vi "S2C_IMAGE_Proc_Timed.vi"(8 "Error In":errorcluster, 10 "DisplayTime":dbl, 11 "ImagePath":path) -> (0 "Error Out":errorcluster)   [LabVIEW 2015]
panel:
  out "Image":picture
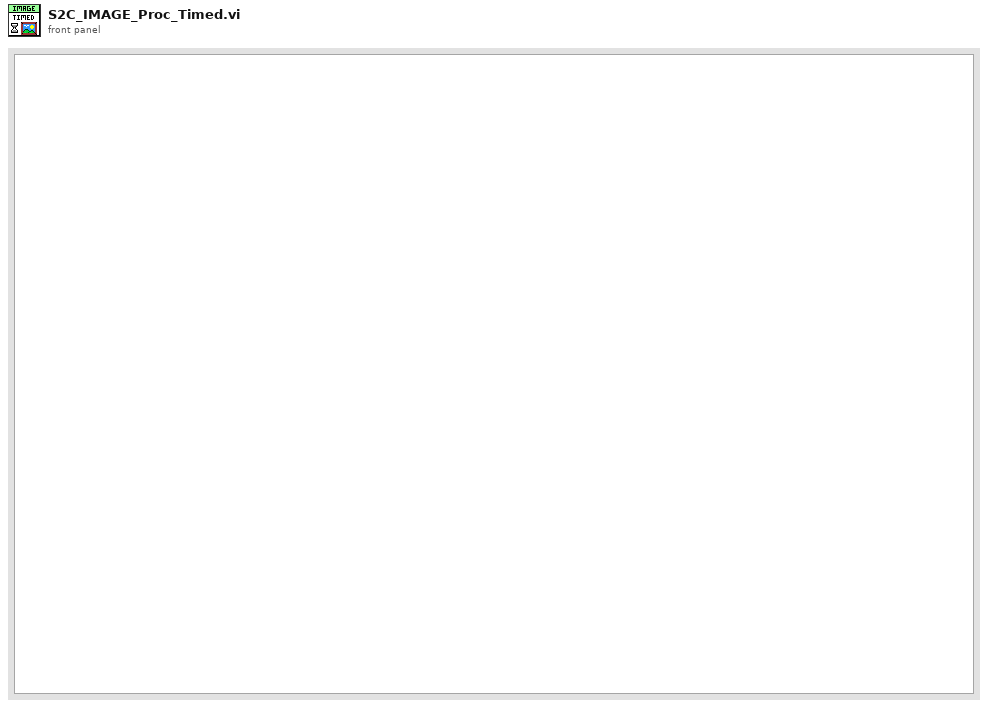
[diagram p1: front panel]
types:
  T1 = cluster{"Left":i16, "Top":i16, "Right":i16, "Bottom":i16}
  T2 = enum32{"Invalid", "Standard", "Closed", "Hidden", "Minimized", "Maximized"}
  T3 = typedef "imagedata.ctl" = cluster{"image type":i32, "image depth":i32, "image":u8[], "mask":u8[], "colors":u32[], "Rectangle":cluster{"left":i16, "top":i16, "right":i16, "bottom":i16}}
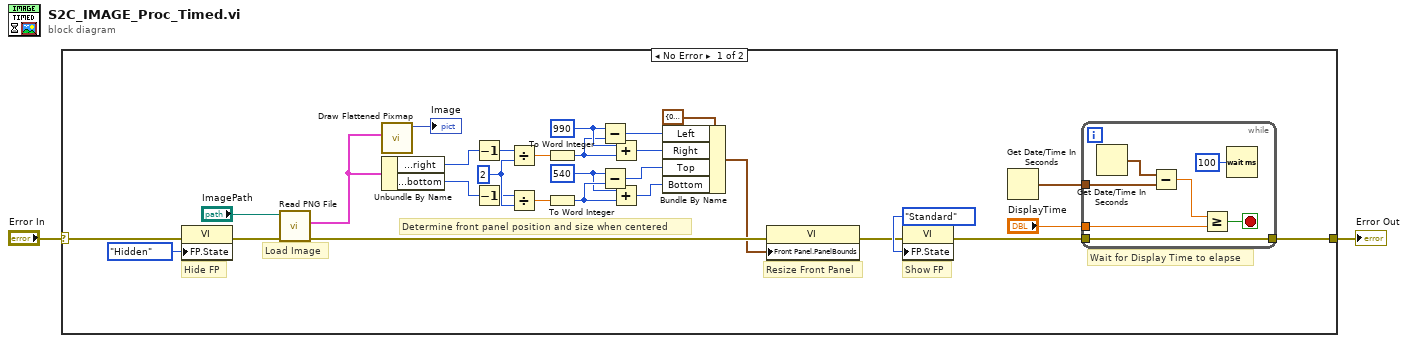
[diagram p0: block diagram]
diagram:
  n1 = case shown="No Error" "Error In" {
    selector: "Error In" -> [w26 w40]
    tunnel: [w30 w40] -> w1
    frame No Error {
      w13 = i16 540
      w16 = i16 990
      w20 = i16 2 ("y")
      # "Show FP"
      # "Resize Front Panel"
      # "Determine front panel position and size when centered"
      # "Hide FP"
      # "Wait for Display Time to elapse"
      # "Load Image"
      n2 = property class="VI"(error in=w26, "FP.State"=T2."Hidden" ("Front Panel Window:State")) -> (error out=w24:errorcluster)  [unwired: 1 in, 1 out]
      n3 = call <vilib>:"Read PNG File.vi"("error in (no error)"=w24, "path to PNG file"="ImagePath") -> ("error out"=w7:errorcluster, "image data"=w27:T3)  [unwired: 7 in, 1 out]
      n4 = call <vilib>:"Draw Flattened Pixmap.vi"("image data"=w27) -> ("new picture"=→"Image":picture)  [unwired: 8 in]
      n5 = Unbundle By Name(w27) -> ("Rectangle.right"=w17:i16, "Rectangle.bottom"=w19:i16)
      n6 = Decrement(x=w17) -> (x-1=w4:i16)
      n7 = Decrement(x=w19) -> (x-1=w3:i16)
      n8 = Divide(x=w4, y=w20) -> (x/y=w18:dbl)
      n9 = Divide(x=w3, y=w20) -> (x/y=w12:dbl)
      n10 = To Word Integer(number=w18) -> (16bit integer=w15:i16)
      n11 = To Word Integer(number=w12) -> (16bit integer=w14:i16)
      n12 = Subtract(x=w16, y=w15) -> (x-y=w11:i16)
      n13 = Subtract(x=w13, y=w14) -> (x-y=w9:i16)
      n14 = Add(x=w16, y=w15) -> (x+y=w10:i16)
      n15 = Add(x=w13, y=w14) -> (x+y=w8:i16)
      n16 = Bundle By Name(cluster=T1 {"Left"=0, "Top"=0, "Right"=0, "Bottom"=0} ("Front Panel Window:Panel Bounds"), "Left"=w11, "Right"=w10, "Top"=w9, "Bottom"=w8) -> (w6:T1)
      n17 = property class="VI"(error in=w7, "Front Panel.PanelBounds"=w6) -> (error out=w22:errorcluster)  [unwired: 1 in, 1 out]
      n18 = property class="VI"(error in=w22, "FP.State"=T2."Standard" ("Front Panel Window:State")) -> (error out=w21:errorcluster)  [unwired: 1 in, 1 out]
      n19 = Get Date/Time In Seconds() -> (seconds since 1Jan1904=w29:timestamp)
      n20 = while {
        tunnel: w21 -> [w39]
        tunnel: [w39] -> w30
        tunnel: w29 -> [w38]
        tunnel: "DisplayTime" -> [w35]
        stop <- w33 stop-if-true
        n21 = Get Date/Time In Seconds() -> (seconds since 1Jan1904=w37:timestamp)
        n22 = Subtract(x=w37, y=w38) -> (x-y=w36:dbl)
        n23 = Greater Or Equal?(x=w36, y=w35) -> (x >= y?=w33:bool)
        n24 = Wait (ms)(milliseconds to wait=u32 100) -> ()  [unwired: 1 out]
      }
    }
    frame Error {
    }
  }
  "Error Out" <- w1
